vi "Post New Data.vi"(8 "error in (no error)":errorcluster, 10 "Data Item":T1) -> (0 "error out":errorcluster)   [LabVIEW 2016, in "Hall Effect Library.lvlib"]
uses:
  Hall Effect Library.lvlib
  Public/Controls/Data Items.ctl
  Public/Controls/Message Types.ctl
  Global Variables/Communication.vi
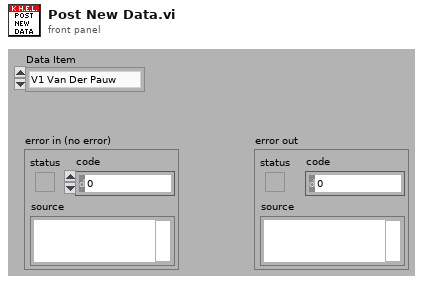
[diagram p1: front panel]
types:
  T1 = typedef "Hall Effect Library.lvlib/Data Items.ctl" = enum16{"V1 Van Der Pauw", "V2 Van Der Pauw", "V3 Van Der Pauw", "V4 Van Der Pauw", "V5 Van Der Pauw", "V6 Van Der Pauw", "V7 Van Der Pauw", "V8 Van Der Pauw", "V1 Hall Effect", "V2 Hall Effect", "V3 Hall Effect", "V4 Hall Effect", "V5 Hall Effect", "V6  Hall Effect", "V7 Hall Effect", "V8 Hall Effect", "V1 Res Bar", "V1 Hall Bar", "V1 Res 6-Cot", "V2 Res 6-Cot", "V3 Res 6-Cot", "V4 Res 6-Cot", "V1 Hall 6-Cot", "V2 Hall 6-Cot", "V3 Hall 6-Cot", "V4 Hall 6-Cot", "V5 Hall 6-Cot", "V6 Hall 6-Cot", "V7 Hall 6-Cot", "V8 Hall 6-Cot", "V1 Res 8-Cot", "V2 Res 8-Cot", "V3 Res 8-Cot", "V4 Res 8-Cot", "V1 Hall 8-Cot", "V2 Hall 8-Cot", "V3 Hall 8-Cot", "V4 Hall 8-Cot", "Van Der Pauw Results", "Hall Effect Results", "Bar Sample Resistivity Results", "Bar Sample Hall Results", "6-Contact Resistivity Results", "6-Contact Hall Results", "8-Contact Resistivity Results", "8-Contact Hall Results"}
  T2 = typedef "Hall Effect Library.lvlib/Message Types.ctl" = enum16{"Status", "New Data", "Test End Normal", "Test End User Abort", "Test End Error"}
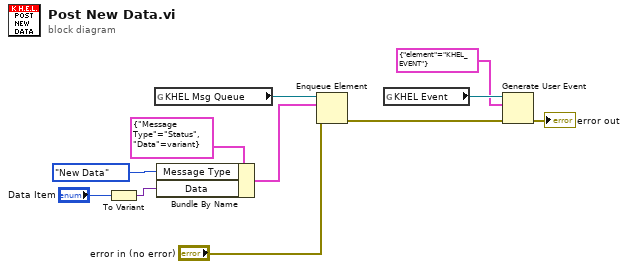
[diagram p0: block diagram]
diagram:
  n1 = To Variant(anything="Data Item") -> (Variant=w9:variant)
  n2 = global read "Communication.vi" "KHEL Msg Queue"() -> (w6:refnum<queue>)
  n3 = Bundle By Name(cluster=cluster{"Message Type":T2, "Data":variant} {"Message Type"=enum."Status", "Data"=variant} ("element"), "Message Type"=Message_Types."New Data", "Data"=w9) -> (w10:cluster{"Message Type":T2, "Data":variant})
  n4 = Enqueue Element(queue=w6, element=w10, error in (no error)="error in (no error)") -> (error out=w3:errorcluster)  [unwired: 3 out]
  n5 = global read "Communication.vi" "KHEL Event"() -> (w2:refnum<user-event>)
  n6 = Generate User Event(user event=w2, event data cluster=cluster{"element":string} {"element"="KHEL_EVENT"}, error in=w3) -> (error out=→"error out":errorcluster)  [unwired: 1 in, 1 out]
